vi "main_picometerControl.vi"() -> ()   [LabVIEW 2018]
uses:
  Device VIs/Verbal.vi
panel:
  out "Motion":bool
  in  "单步时间ms":u32=100
  in  "CH2归0":bool
  in  "CH1归0":bool
  out "OK":bool
  in  "制动":bool
  in  "CH2启动":bool
  in  "CH1启动":bool
  in  "CH2 运动步数":i32
  in  "CH1 运动步数":i32
  out "CH2 当前位置":i32
  out "CH1 当前位置":i32
  out "状态":string
  out "error out":errorcluster
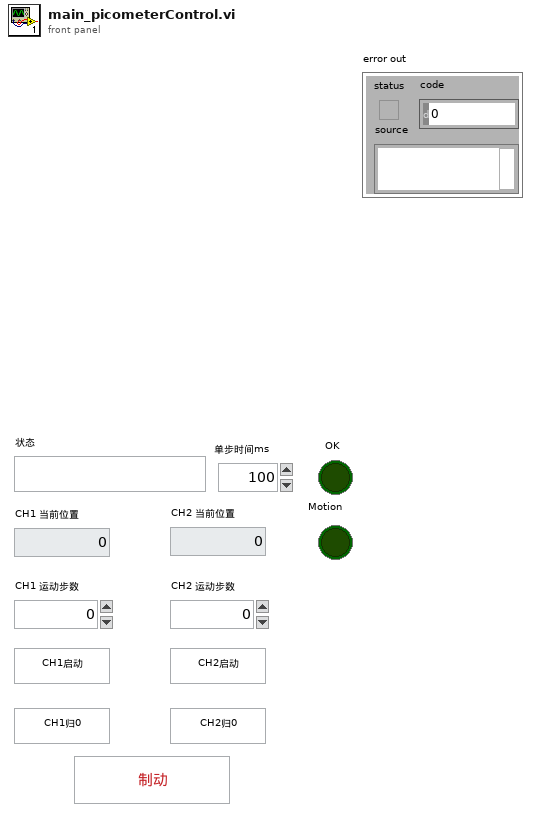
[diagram p1: front panel]
types:
  T1 = cluster{"DeviceKey":string, "Device Address":i32, "Controller Name":string}[]
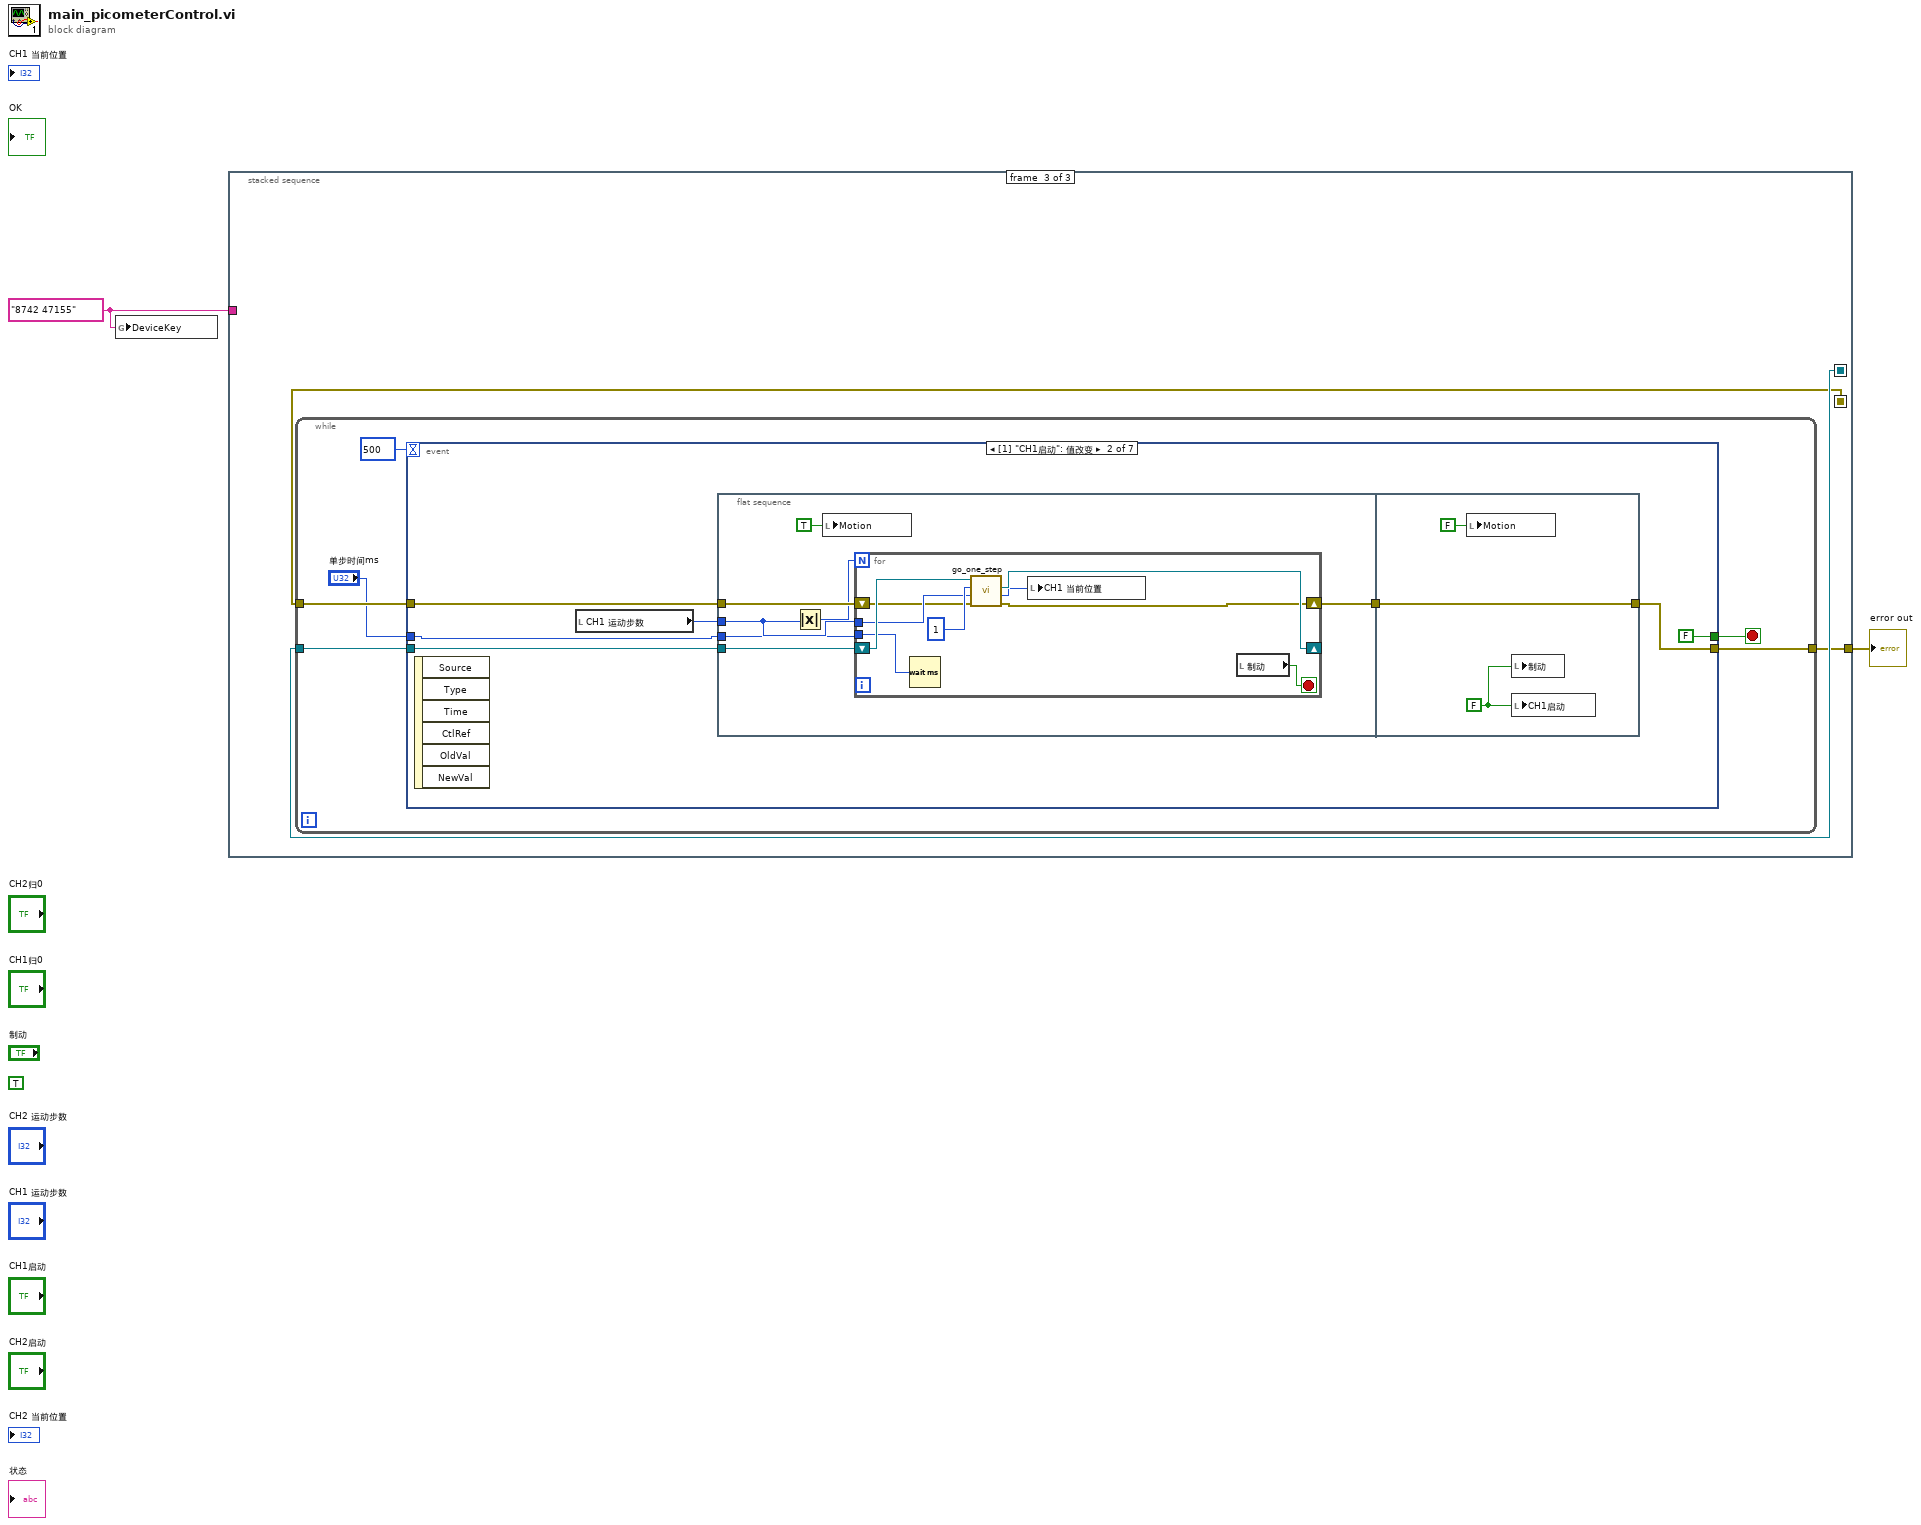
[diagram p0: block diagram]
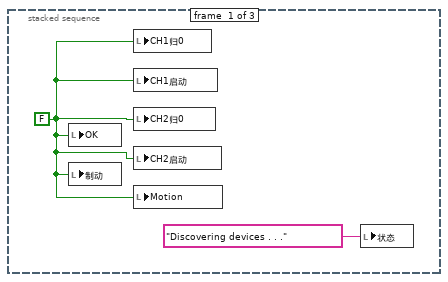
[diagram p2: hidden frame]
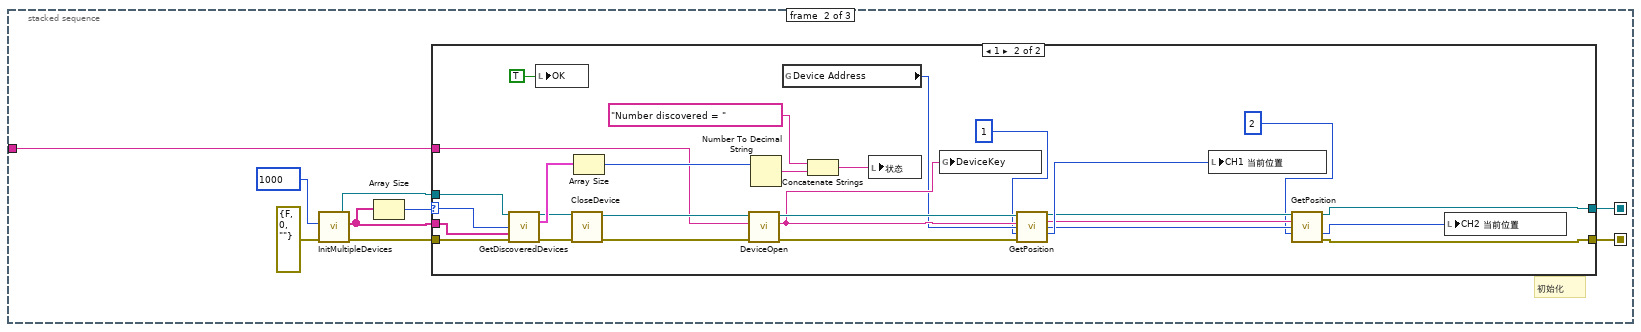
[diagram p3: hidden frame]
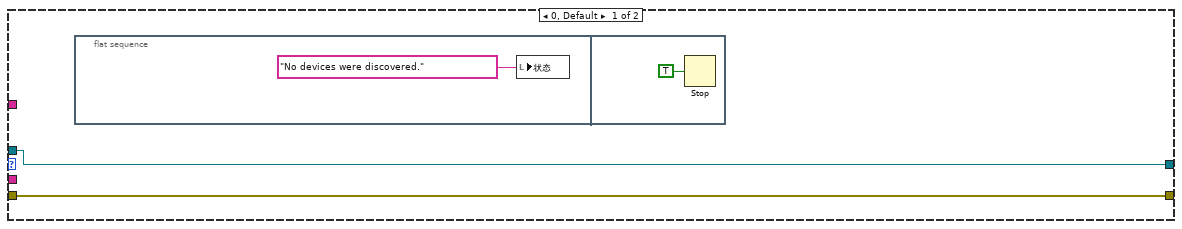
[diagram p4: hidden frame]
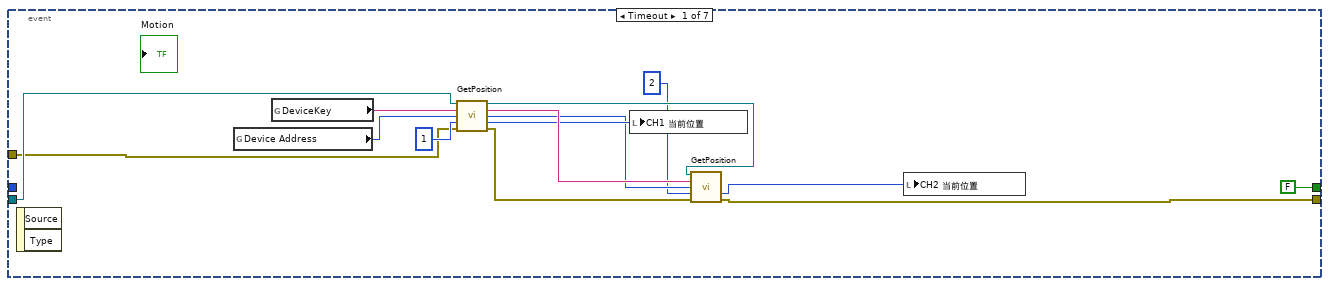
[diagram p5: hidden frame]
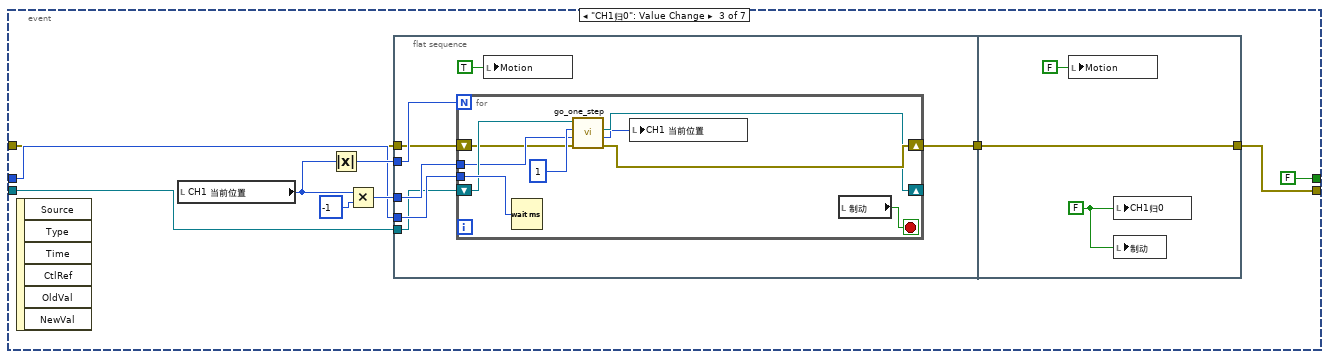
[diagram p6: hidden frame]
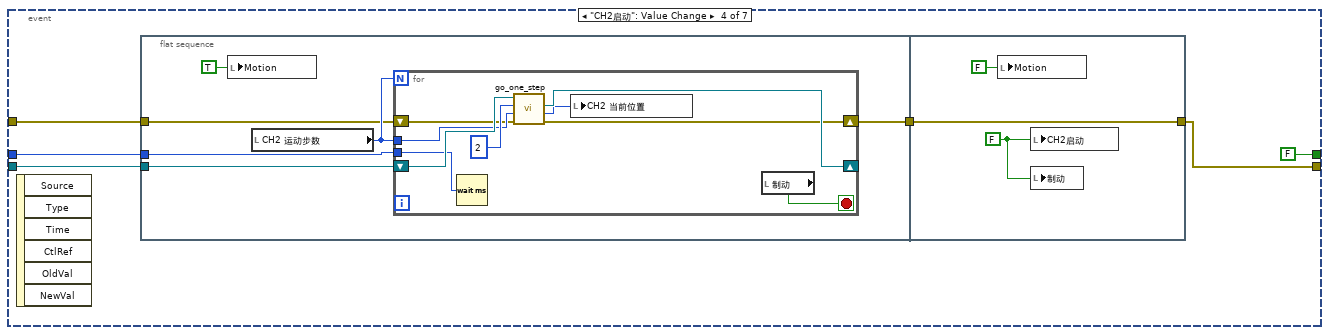
[diagram p7: hidden frame]
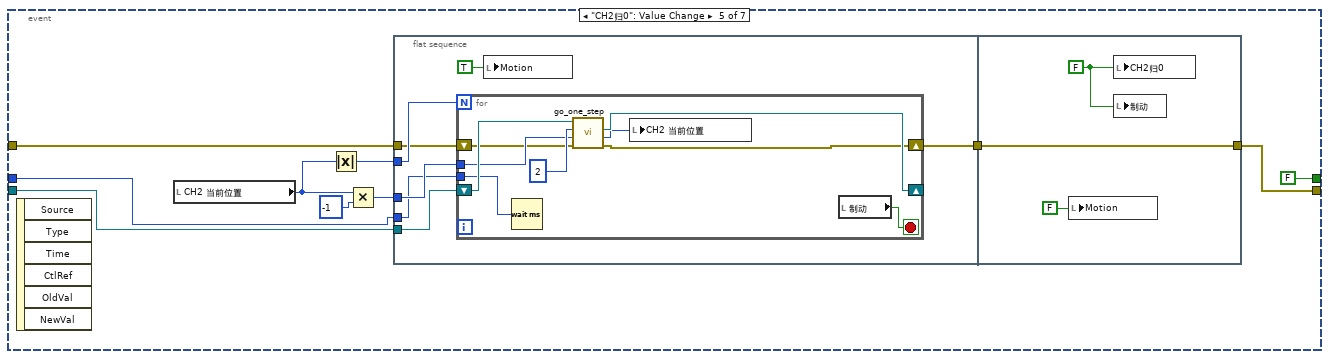
[diagram p8: hidden frame]
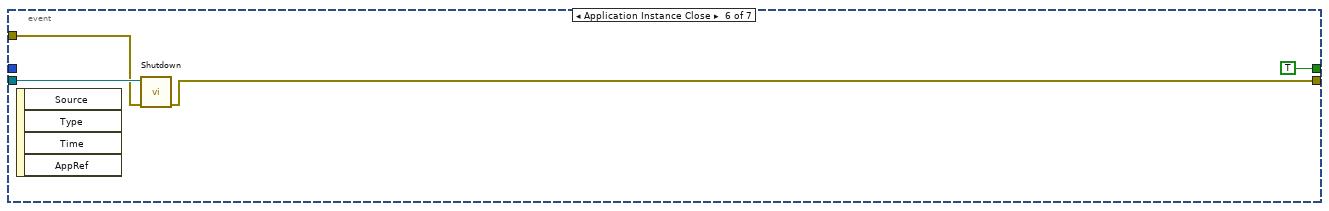
[diagram p9: hidden frame]
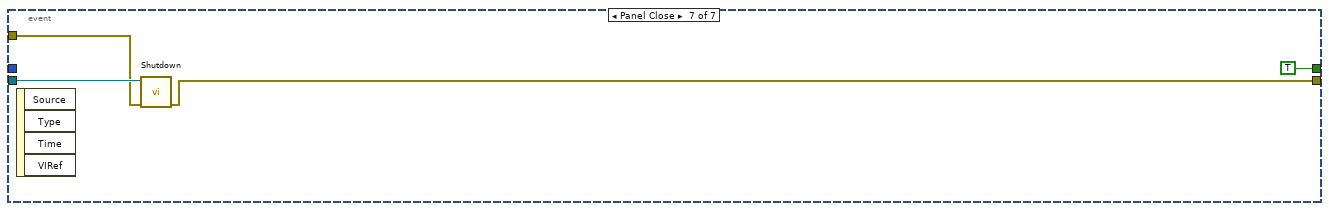
[diagram p10: hidden frame]
diagram:
  (unwired) TRUE
  w2 = "8742 47155" ("Message")
  n1 = global write "Verbal.vi" "DeviceKey"(w2) -> ()
  n2 = stacked-sequence {
    seq-local: [_ w6 _] -> [_ _ w48]
    seq-local: [_ w5 _] -> [_ _ w47]
    tunnel: w2 -> [_ w7 _]
    tunnel: [_ _ w46] -> w1
    frame #0 {
      w3 = FALSE ("Motion")
      n3 = local write "OK"(w3) -> ()
      n4 = local write "制动"(w3) -> ()
      n5 = local write "CH1归0"(w3) -> ()
      n6 = local write "CH1启动"(w3) -> ()
      n7 = local write "CH2归0"(w3) -> ()
      n8 = local write "CH2启动"(w3) -> ()
      n9 = local write "Motion"(w3) -> ()
      n10 = local write "状态"("Discovering devices . . ." ("Message")) -> ()
    }
    frame #1 {
      # "初始化"
      n11 = call "InitMultipleDevices.vi"("error in (no error)"=errorcluster {"status"=FALSE, "code"=0, "source"=""}, "msecDelayForDiscovery"=1000) -> ("error out"=w8:errorcluster, "DeviceKey List Out"=w9:string[], "CmdLib Out"=w10:refnum<k24>)  [unwired: 3 in]
      n12 = Array Size(array=w9) -> (size(s)=w11:i32)
      n13 = case shown="1" w11 {
        selector: w11 -> [_ w41]
        tunnel: w10 -> [w15 w42]
        tunnel: w9 -> [_ w40]
        tunnel: w8 -> [w14 w39]
        tunnel: w7 -> [_ w35]
        tunnel: [w15 w21] -> w6
        tunnel: [w14 w19] -> w5
        frame 0, Default {
          n14 = flat-sequence {
            frame #0 {
              n15 = local write "状态"("No devices were discovered." ("Input String")) -> ()
            }
            frame #1 {
              n16 = Stop(stop? (T)=TRUE ("停止？(T)")) -> ()
            }
          }
        }
        frame 1 {
          n17 = call "GetDiscoveredDevices.vi"("CmdLib In"=w42, "Master Count"=w41, "DeviceKey List"=w40, "error in"=w39) -> ("CmdLib Out"=w37:refnum<k24>, "Device Array"=w38:T1, "error out"=w34:errorcluster)  [unwired: 9 in]
          n18 = local write "OK"(TRUE ("等待指令")) -> ()
          n19 = call "CloseDevice.vi"("error in"=w34, "CmdLib In"=w37) -> ("error out"=w33:errorcluster, "CmdLib Out"=w36:refnum<k24>)  [unwired: 8 in]
          n20 = Array Size(array=w38) -> (size(s)=w45:i32)
          n21 = call "DeviceOpen.vi"("error in (no error)"=w33, "DeviceKey In"=w35, "CmdLib In"=w36) -> ("error out"=w28:errorcluster, "DeviceKey Out"=w31:string, "CmdLib Out"=w32:refnum<k24>)  [unwired: 2 in]
          n22 = Number To Decimal String(number=w45) -> (decimal integer string=w43:string)  [unwired: 1 in]
          n23 = global read "Verbal.vi" "Device Address"() -> (w30:i32)
          n24 = Concatenate Strings("Number discovered = " ("string"), w43) -> (w20:string)
          n25 = local write "状态"(w20) -> ()
          n26 = global write "Verbal.vi" "DeviceKey"(w31) -> ()
          n27 = call "GetPosition.vi"("CmdLib In"=w32, "DeviceKey In"=w31, "Device Address In"=w30, "Motor"=1, "error in (no error)"=w28) -> ("CmdLib Out"=w26:refnum<k24>, "DeviceKey Out"=w25:string, "Device Address Out"=w24:i32, "Position"=w27:i32)  [unwired: 6 in, 1 out]
          n28 = local write "CH1 当前位置"(w27) -> ()
          n29 = call "GetPosition.vi"("CmdLib In"=w26, "DeviceKey In"=w25, "Device Address In"=w24, "Motor"=2) -> ("CmdLib Out"=w21:refnum<k24>, "Position"=w22:i32, "error out"=w19:errorcluster)  [unwired: 7 in, 2 out]
          n30 = local write "CH2 当前位置"(w22) -> ()
        }
      }
    }
    frame #2 {
      n31 = while {
        tunnel: w48 -> [w53]
        tunnel: w47 -> [w52]
        tunnel: [w51] -> w46
        stop <- w50 stop-if-true
        n32 = event shown="[1] \"CH1启动\": 值改变" {
          selector: _ -> [_ _ _ _ _ _ _]
          dyn-events: _ -> [_ _ _ _ _ _ _]
          timeout: 500 -> [_ _ _ _ _ _ _]
          tunnel: w53 -> [w68 w75 w99 w129 w153 w180 w184]
          tunnel: w52 -> [w57 w74 w98 w127 w152 w179 w183]
          tunnel: [w55 w73 w96 w128 w151 w178 w182] -> w51
          tunnel: [FALSE FALSE FALSE FALSE FALSE TRUE TRUE] -> w50
          tunnel: "单步时间ms" -> [_ w70 w100 w125 w149 _ _]
          event Timeout {
            n33 = event-data() -> ()  [unwired: 1 in, 2 out]
            n34 = global read "Verbal.vi" "Device Address"() -> (w66:i32)
            n35 = global read "Verbal.vi" "DeviceKey"() -> (w67:string)
            n36 = call "GetPosition.vi"("CmdLib In"=w68, "DeviceKey In"=w67, "Device Address In"=w66, "Motor"=1, "error in (no error)"=w57) -> ("CmdLib Out"=w64:refnum<k24>, "DeviceKey Out"=w63:string, "Device Address Out"=w61:i32, "Position"=w62:i32, "error out"=w56:errorcluster)  [unwired: 6 in]
            n37 = local write "CH1 当前位置"(w62) -> ()
            n38 = call "GetPosition.vi"("CmdLib In"=w64, "DeviceKey In"=w63, "Device Address In"=w61, "Motor"=2, "error in (no error)"=w56) -> ("Position"=w59:i32, "error out"=w55:errorcluster)  [unwired: 6 in, 3 out]
            n39 = local write "CH2 当前位置"(w59) -> ()
          }
          event "CH1启动": Value Change {
            n40 = event-data() -> ()  [unwired: 1 in, 6 out]
            n41 = local read "CH1 运动步数"() -> (w71:i32)
            n42 = flat-sequence {
              tunnel: w75 -> [w82]
              tunnel: w74 -> [w81]
              tunnel: w71 -> [w78]
              tunnel: w70 -> [w77]
              tunnel: [w80] -> w69
              tunnel: [w94] -> w73
              tunnel: w69 -> [w94]
              frame #0 {
                n43 = Absolute Value(x=w78) -> (abs(x)=w79:i32)
                n44 = local write "Motion"(TRUE ("Motion")) -> ()
                n45 = for {
                  N: w79 -> [_]
                  shift-right: [w85] -> w80
                  shift-left: w81 -> [w87]
                  shift-right: [w90] -> _
                  shift-left: w82 -> [w91]
                  tunnel: w78 -> [w88]
                  tunnel: w77 -> [w84]
                  stop <- w83 stop-if-true
                  n46 = Wait (ms)(milliseconds to wait=w84) -> ()  [unwired: 1 out]
                  n47 = call "go_one_step.vi"("error in"=w87, "Step"=w88, "Motor"=1, "CmdLib In"=w91) -> ("error out"=w85:errorcluster, "Position"=w86:i32, "CmdLib Out"=w90:refnum<k24>)  [unwired: 1 in]
                  n48 = local write "CH1 当前位置"(w86) -> ()
                  n49 = local read "制动"() -> (w83:bool)
                }
              }
              frame #1 {
                w93 = FALSE ("制动")
                n50 = local write "Motion"(FALSE ("Motion")) -> ()
                n51 = local write "制动"(w93) -> ()
                n52 = local write "CH1启动"(w93) -> ()
              }
            }
          }
          event "CH1归0": Value Change {
            n53 = event-data() -> ()  [unwired: 1 in, 6 out]
            n54 = local read "CH1 当前位置"() -> (w103:i32)
            n55 = Absolute Value(x=w103) -> (abs(x)=w104:i32)
            n56 = Multiply(x=w103, y=-1) -> (x*y=w101:i32)
            n57 = flat-sequence {
              tunnel: w104 -> [w111]
              tunnel: w101 -> [w110]
              tunnel: w100 -> [w109]
              tunnel: w99 -> [w108]
              tunnel: w98 -> [w107]
              tunnel: [w106] -> w95
              tunnel: [w123] -> w96
              tunnel: w95 -> [w123]
              frame #0 {
                n58 = for {
                  N: w111 -> [_]
                  tunnel: w110 -> [w117]
                  tunnel: w109 -> [w120]
                  shift-right: [w115] -> w106
                  shift-left: w107 -> [w116]
                  shift-right: [w114] -> _
                  shift-left: w108 -> [w119]
                  stop <- w112 stop-if-true
                  n59 = Wait (ms)(milliseconds to wait=w120) -> ()  [unwired: 1 out]
                  n60 = call "go_one_step.vi"("error in"=w116, "Step"=w117, "Motor"=1, "CmdLib In"=w119) -> ("error out"=w115:errorcluster, "Position"=w113:i32, "CmdLib Out"=w114:refnum<k24>)  [unwired: 1 in]
                  n61 = local write "CH1 当前位置"(w113) -> ()
                  n62 = local read "制动"() -> (w112:bool)
                }
                n63 = local write "Motion"(TRUE ("Motion")) -> ()
              }
              frame #1 {
                w122 = FALSE ("制动")
                n64 = local write "Motion"(FALSE ("Motion")) -> ()
                n65 = local write "CH1归0"(w122) -> ()
                n66 = local write "制动"(w122) -> ()
              }
            }
          }
          event "CH2启动": Value Change {
            n67 = event-data() -> ()  [unwired: 1 in, 6 out]
            n68 = flat-sequence {
              tunnel: w129 -> [w135]
              tunnel: w127 -> [w132]
              tunnel: w125 -> [w131]
              tunnel: [w133] -> w124
              tunnel: [w147] -> w128
              tunnel: w124 -> [w147]
              frame #0 {
                n69 = local write "Motion"(TRUE ("Motion")) -> ()
                n70 = local read "CH2 运动步数"() -> (w134:i32)
                n71 = for {
                  N: w134 -> [_]
                  tunnel: w134 -> [w142]
                  shift-right: [w141] -> _
                  shift-left: w135 -> [w144]
                  shift-right: [w139] -> w133
                  shift-left: w132 -> [w138]
                  tunnel: w131 -> [w137]
                  stop <- w136 stop-if-true
                  n72 = Wait (ms)(milliseconds to wait=w137) -> ()  [unwired: 1 out]
                  n73 = call "go_one_step.vi"("error in"=w138, "Step"=w142, "Motor"=2, "CmdLib In"=w144) -> ("error out"=w139:errorcluster, "Position"=w140:i32, "CmdLib Out"=w141:refnum<k24>)  [unwired: 1 in]
                  n74 = local write "CH2 当前位置"(w140) -> ()
                  n75 = local read "制动"() -> (w136:bool)
                }
              }
              frame #1 {
                w146 = FALSE
                n76 = local write "Motion"(FALSE ("Motion")) -> ()
                n77 = local write "CH2启动"(w146) -> ()
                n78 = local write "制动"(w146) -> ()
              }
            }
          }
          event "CH2归0": Value Change {
            n79 = event-data() -> ()  [unwired: 1 in, 6 out]
            n80 = local read "CH2 当前位置"() -> (w156:i32)
            n81 = Absolute Value(x=w156) -> (abs(x)=w157:i32)
            n82 = Multiply(x=w156, y=-1) -> (x*y=w154:i32)
            n83 = flat-sequence {
              tunnel: w157 -> [w164]
              tunnel: w154 -> [w163]
              tunnel: w153 -> [w162]
              tunnel: w152 -> [w161]
              tunnel: w149 -> [w159]
              tunnel: [w160] -> w148
              tunnel: [w176] -> w151
              tunnel: w148 -> [w176]
              frame #0 {
                n84 = for {
                  N: w164 -> [_]
                  tunnel: w163 -> [w170]
                  shift-right: [w172] -> _
                  shift-left: w162 -> [w173]
                  shift-right: [w168] -> w160
                  shift-left: w161 -> [w169]
                  tunnel: w159 -> [w166]
                  stop <- w165 stop-if-true
                  n85 = Wait (ms)(milliseconds to wait=w166) -> ()  [unwired: 1 out]
                  n86 = call "go_one_step.vi"("error in"=w169, "Step"=w170, "Motor"=2, "CmdLib In"=w173) -> ("error out"=w168:errorcluster, "Position"=w167:i32, "CmdLib Out"=w172:refnum<k24>)  [unwired: 1 in]
                  n87 = local write "CH2 当前位置"(w167) -> ()
                  n88 = local read "制动"() -> (w165:bool)
                }
                n89 = local write "Motion"(TRUE ("Motion")) -> ()
              }
              frame #1 {
                w175 = FALSE ("制动")
                n90 = local write "Motion"(FALSE ("Motion")) -> ()
                n91 = local write "CH2归0"(w175) -> ()
                n92 = local write "制动"(w175) -> ()
              }
            }
          }
          event Application Instance Close {
            n93 = event-data() -> ()  [unwired: 1 in, 4 out]
            n94 = call "Shutdown.vi"("error in (no error)"=w179, "CmdLib In"=w180) -> ("error out"=w178:errorcluster)  [unwired: 4 in, 1 out]
          }
          event Panel Close {
            n95 = event-data() -> ()  [unwired: 1 in, 4 out]
            n96 = call "Shutdown.vi"("error in (no error)"=w183, "CmdLib In"=w184) -> ("error out"=w182:errorcluster)  [unwired: 4 in, 1 out]
          }
        }
      }
    }
  }
  "error out" <- w1
